vi "CC Hardware Config Editor.vi"() -> ()   [LabVIEW 2020]
panel:
  in  "Close":bool
  in  "Add Device":bool
  in  "Add Type":bool
  in  "System Setup":string(tree)
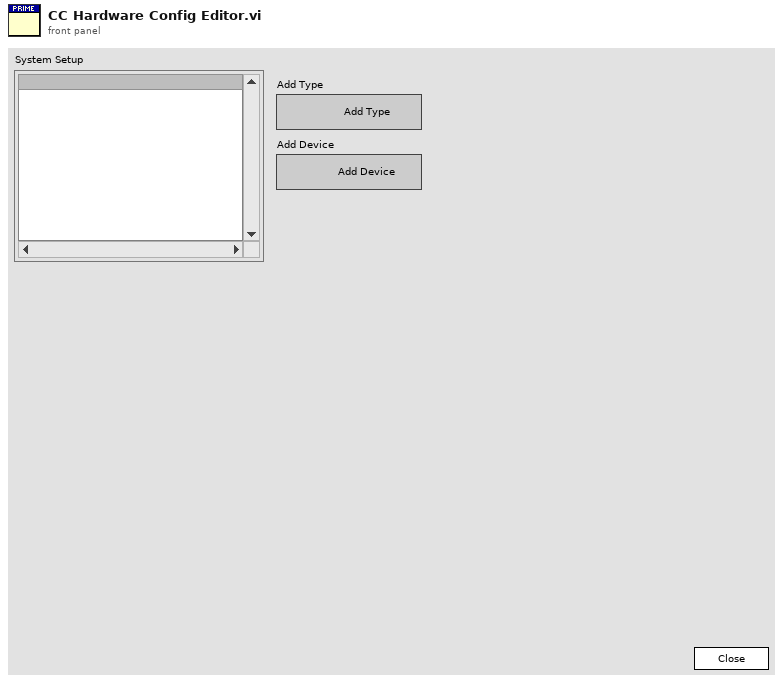
[diagram p1: front panel]
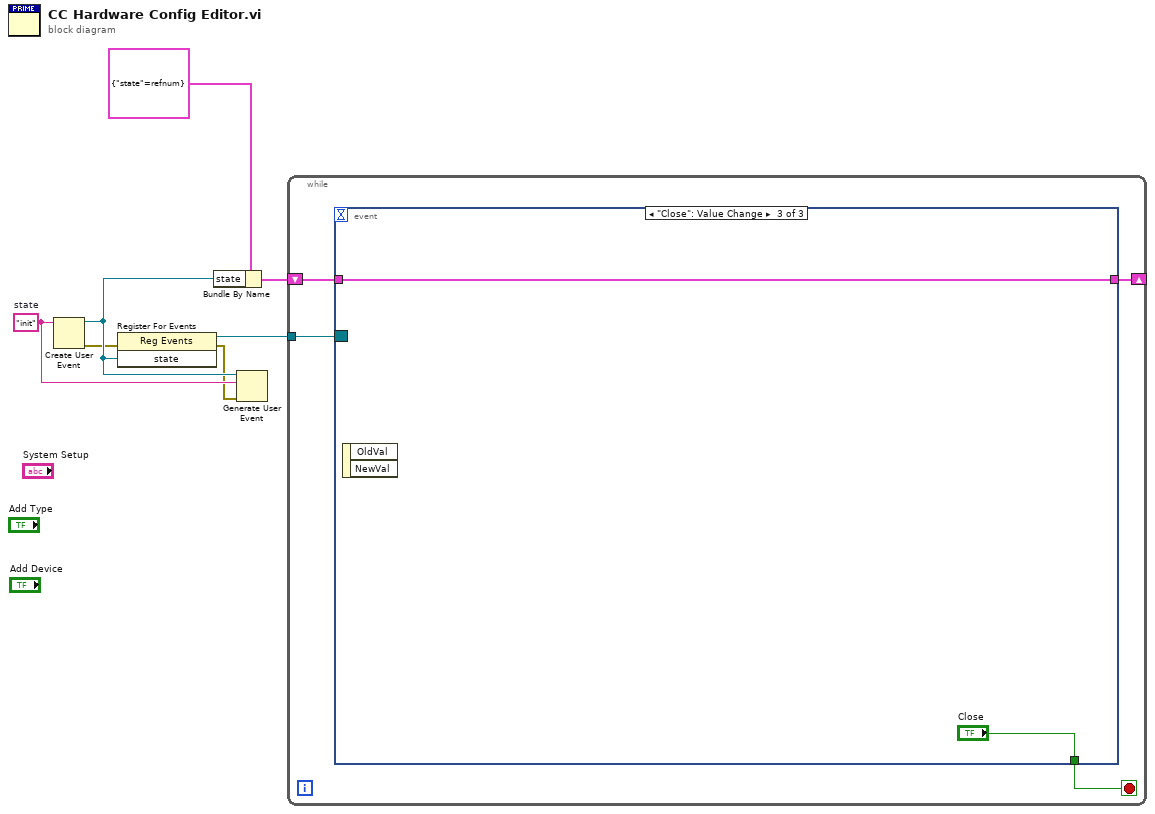
[diagram p0: block diagram]
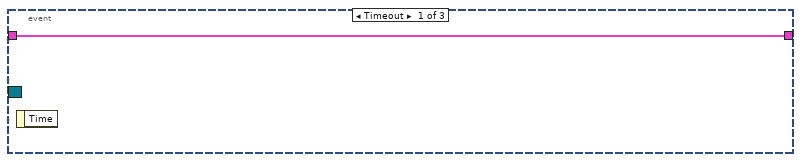
[diagram p2: hidden frame]
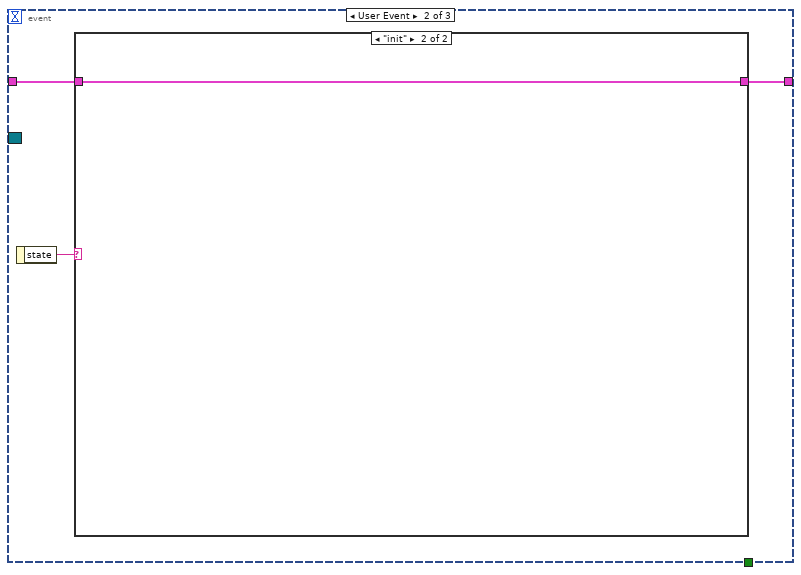
[diagram p3: hidden frame]
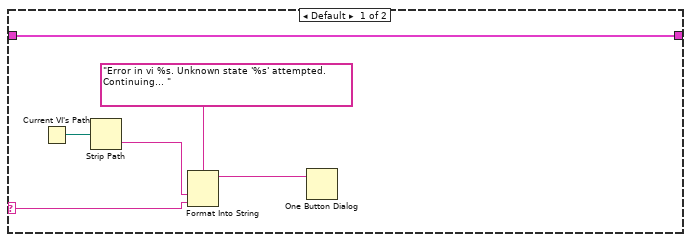
[diagram p4: hidden frame]
diagram:
  w3 = "init"  # state
  n1 = Create User Event(user event datatype=w3) -> (user event=w5:refnum<user-event>, error out=w1:errorcluster)  [unwired: 1 in]
  n2 = register-events(error in=w1, w5) -> (reference out=w4:refnum<event-registration>, error out=w2:errorcluster)  [unwired: 1 in]
  n3 = Bundle By Name(cluster=cluster{"state":refnum<user-event>} {"state"=refnum}, "state"=w5) -> (w6:cluster{"state":refnum<user-event>})
  n4 = Generate User Event(user event=w5, event data cluster=w3, error in=w2) -> ()  [unwired: 1 in, 2 out]
  n5 = while {
    tunnel: w4 -> [w11]
    shift-right: [w9] -> _
    shift-left: w6 -> [w10]
    stop <- w8 stop-if-true
    n6 = event shown="[2] \"Close\": Value Change" {
      selector: w11 -> [_ _ _]
      dyn-events: _ -> [_ _ _]
      timeout: _ -> [_ _ _]
      tunnel: w10 -> [w12 w14 w24]
      tunnel: [w12 w13 w24] -> w9
      tunnel: [_ _ "Close"] -> w8
      event Timeout {
        n7 = event-data() -> ()  [unwired: 1 in, 1 out]
      }
      event User Event {
        n8 = event-data() -> ("state"=w15:string)  [unwired: 1 in]
        n9 = case shown="\"init\"" w15 {
          selector: w15 -> [w20 _]
          tunnel: w14 -> [w16 w22]
          tunnel: [w16 w22] -> w13
          frame Default {
            n10 = Current VI's Path() -> (path=w19:path)
            n11 = Strip Path(path=w19) -> (name=w18:string)  [unwired: 1 out]
            n12 = Format Into String(format string="Error in vi %s. Unknown state '%s' attempted. Continuing... ", w18, w20) -> (resulting string=w17:string)  [unwired: 2 in, 1 out]
            n13 = One Button Dialog(message=w17) -> ()  [unwired: 1 in, 1 out]
          }
          frame "init" {
          }
        }
      }
      event "Close": Value Change {
        n14 = event-data() -> ()  [unwired: 1 in, 2 out]
      }
    }
  }
